vi "scope_viewer.vi"() -> ()   [LabVIEW 2019]
uses:
  <instrlib>/niScope/Controls/niScope trigger source.ctl
  <instrlib>/niScope/Controls/niScope trigger coupling.ctl
  <instrlib>/niScope/Controls/niScope trigger slope.ctl
  <instrlib>/niScope/Controls/niScope vertical coupling.ctl
  <vilib>/Waveform/WDTOps.llb/WDT Align Waveform Timestamps DBL.vi
  <vilib>/Waveform/WDTFileIO.llb/Export Waveform To Spreadsheet File.vi
  <instrlib>/niScope/Acquire/Fetch/niScope Fetch WDT.vi
  <instrlib>/niScope/Configure/Trigger/niScope Configure Trigger Edge.vi
  <vilib>/regexp/Match Regular Expression.xnode
panel:
  in  "Tab Control":T1(tab)
  in  "C1 vertical coupling":T2=1 caption="vertical coupling" items=["AC", "DC", "Ground"]
  in  "C1 probe attenuation":dbl=1.0 caption="probe attenuation" format="%.1f"
  in  "C1 vertical range":dbl=5.0 caption="vertical range" min=0.1 max=5.0 step=0.1 format="%.2f"
  in  "C1 vertical offset":dbl caption="vertical offset" format="%.4f"
  in  "C1 enabled":bool=TRUE caption="Enabled?"
  in  "C1 maximum input frequency":dbl caption="max input frequency" format="%.2f"
  in  "C1 input impedance":u32(ring) caption="input impedance" items=["1 mega ohm"=0, "50 ohms"=2]
  in  "C2 enabled":bool=TRUE caption="Enabled?"
  in  "C2 input impedance":u32(ring) caption="input impedance" items=["1 mega ohm"=0, "50 ohms"=2]
  in  "C2 maximum input frequency":dbl caption="max input frequency" format="%.2f"
  in  "C2 vertical coupling":T2=1 caption="vertical coupling" items=["AC", "DC", "Ground"]
  in  "C2 probe attenuation":dbl=1.0 caption="probe attenuation" format="%.1f"
  in  "C2 vertical range":dbl=5.0 caption="vertical range" min=0.1 max=5.0 step=0.1 format="%.2f"
  in  "C2 vertical offset":dbl caption="vertical offset" format="%.4f"
  in  "Num Trace":dbl=1.0 min=1.0 step=1.0
  in  "Summed/Average":u16(ring) items=["Average", "Summed"]
  in  "Trigger delay":dbl caption="trigger delay" format="%.4f"
  in  "Trigger slope":T3 items=["Positive", "Negative"]
  in  "Trigger level":dbl=0.5
  in  "Trigger coupling":T4=1 caption="C1 trigger coupling" items=["AC"=0, "DC"=1, "HF Reject"=3, "LF Reject"=4, "AC Plus HF Reject"=1001]
  in  "Trigger source":T5="0" caption="Source"
  out "Aqusition Time / ms":u32
  out "Aquisition Frequency / Hz":dbl
  in  "tmax (\\mu s)":dbl
  in  "Samples":i64(ring) items=["500 S"=500, "1 kS"=1000, "5 kS"=5000, "10 kS"=10000, "100 kS"=100000, "500 kS"=500000, "1 MS"=1000000, "2.5 MS"=2500000, "5MS"=5000000, "10 MS"=10000000, "20 MS"=20000000]
  in  "Scope Channel":refnum<k15> caption="resource name"
  in  "stop":bool
  in  "Enforce realtime":bool=TRUE caption="enforce realtime"
  in  "Save Scope Conditions":bool
  in  "Load Scope Conditions":bool
  in  "waveforms out 2":waveform(dbl)[](array[waveform])
  in  "Tab Control 2":T6(tab)
  in  "Tab Control 3":enum32{"Channel 1", "Channel 2"}(tab)
  out "Channel 1 Raw":waveform(dbl)(graph)
  out "Channel 2 Raw":waveform(dbl)(graph)
  in  "Tab Control 4":enum32{"Channel 1", "Channel 2"}(tab)
  out "Channel 1 RT avg":waveform(dbl)(graph)
  out "Channel 2 RT avg":waveform(dbl)(graph)
  in  "Tab Control 5":enum32{"Channel 1", "Channel 2"}(tab)
  out "Channel 1 summed":waveform(dbl)(graph)
  out "Channel 2 summed":waveform(dbl)(graph)
  # "Scope Controls"
  # "Channel Enabled?"
  # "Channel Enabled?"
  # "Scope Conditions:"
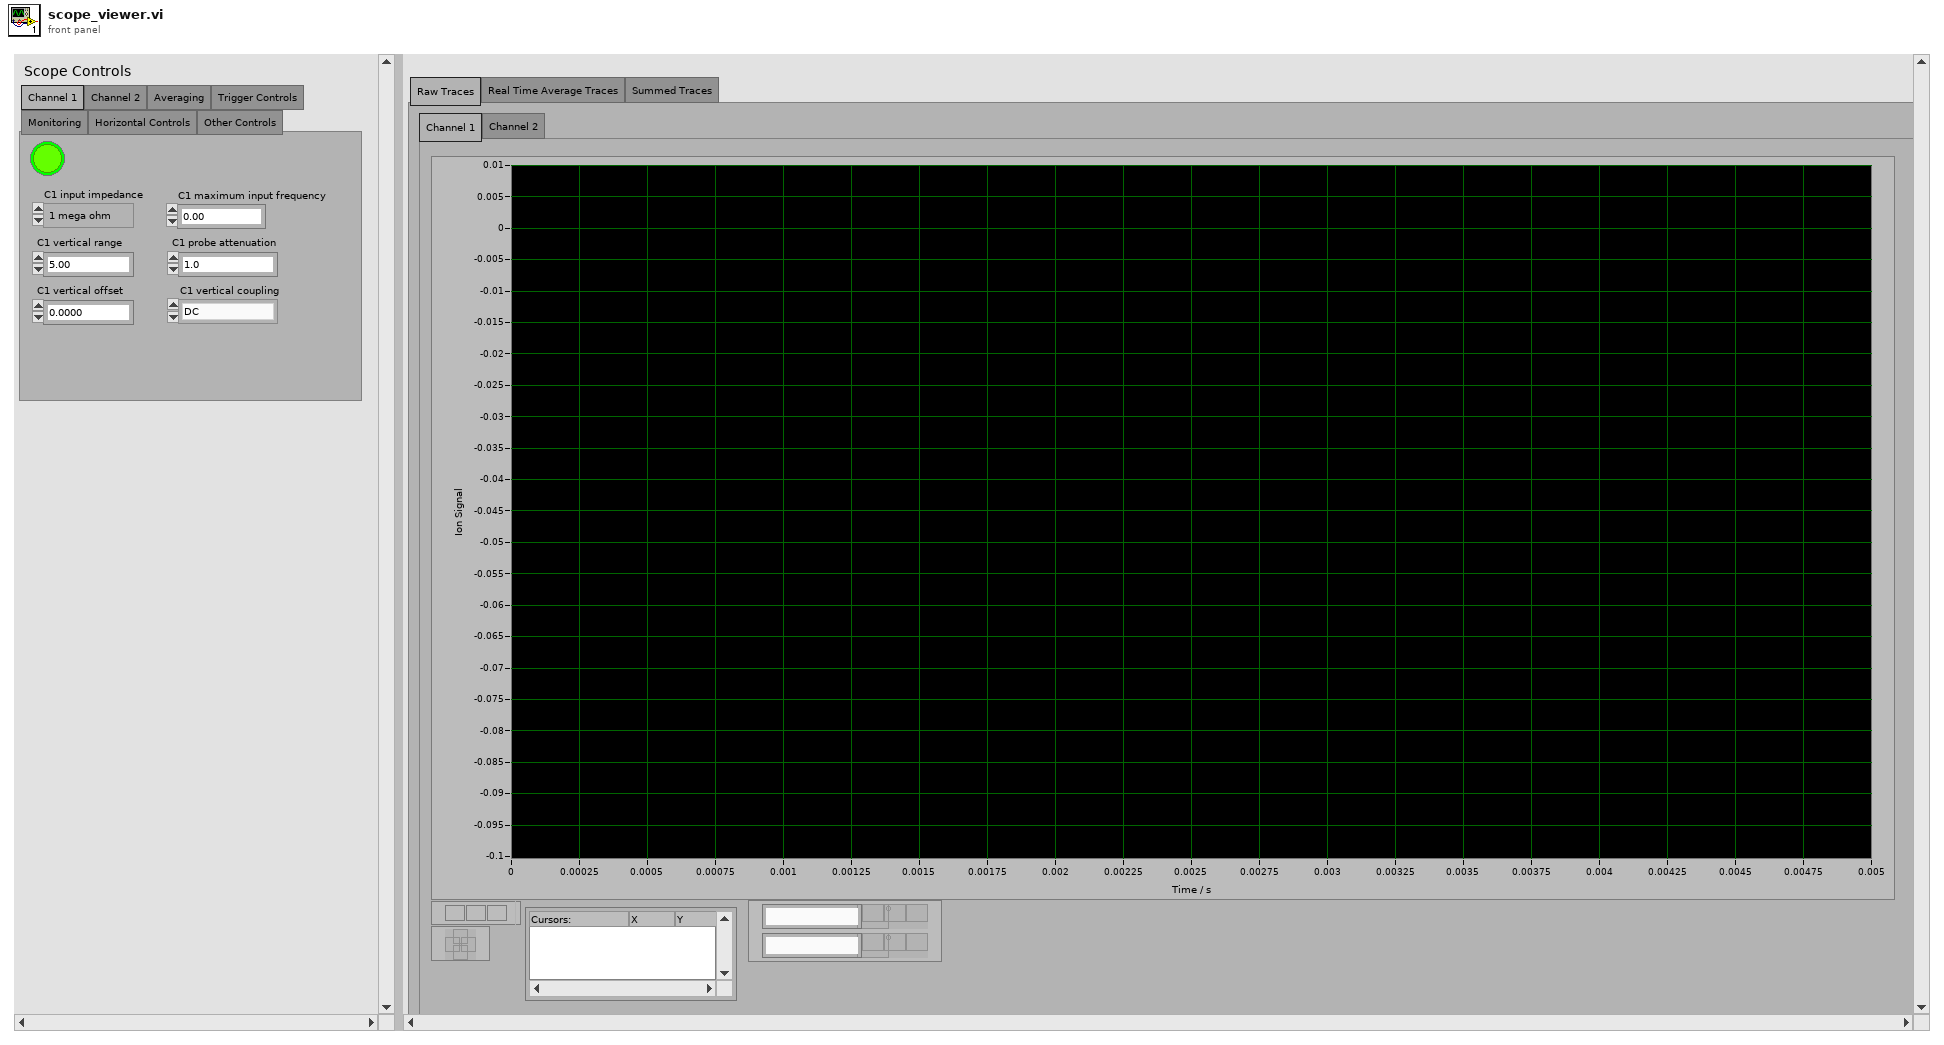
[diagram p1: front panel]
types:
  T1 = enum32{"Channel 1", "Channel 2", "Averaging", "Trigger Controls", "Monitoring", "Horizontal Controls", "Other Controls"}
  T2 = typedef "niScope vertical coupling.ctl" = i32
  T3 = typedef "niScope trigger slope.ctl" = i32
  T4 = typedef "niScope trigger coupling.ctl" = u16
  T5 = typedef "niScope trigger source.ctl" = string
  T6 = enum32{"Raw Traces", "Real Time Average Traces", "Summed Traces"}
  T7 = cluster{"C2 vertical offset":dbl, "C2 vertical range":dbl, "C2 probe attenuation":dbl, "C2 vertical coupling":T2, "C2 maximum input frequency":dbl, "C2 input impedance":u32, "C2 enabled":bool, "C1 input impedance":u32, "C1 maximum input frequency":dbl, "C1 enabled":bool, "C1 vertical offset":dbl, "C1 vertical range":dbl, "C1 probe attenuation":dbl, "C1 vertical coupling":T2, "Samples":i64, "tmax (\\mu s) ":dbl, "Trigger source":T5, "Trigger coupling":T4, "Trigger level":dbl, "Trigger slope":T3, "Trigger delay":dbl, "Enforce realtime":bool, "Aquisition Frequency / Hz":dbl, "Aqusition Time / ms":u32, "Scope Channel":refnum<k15>}
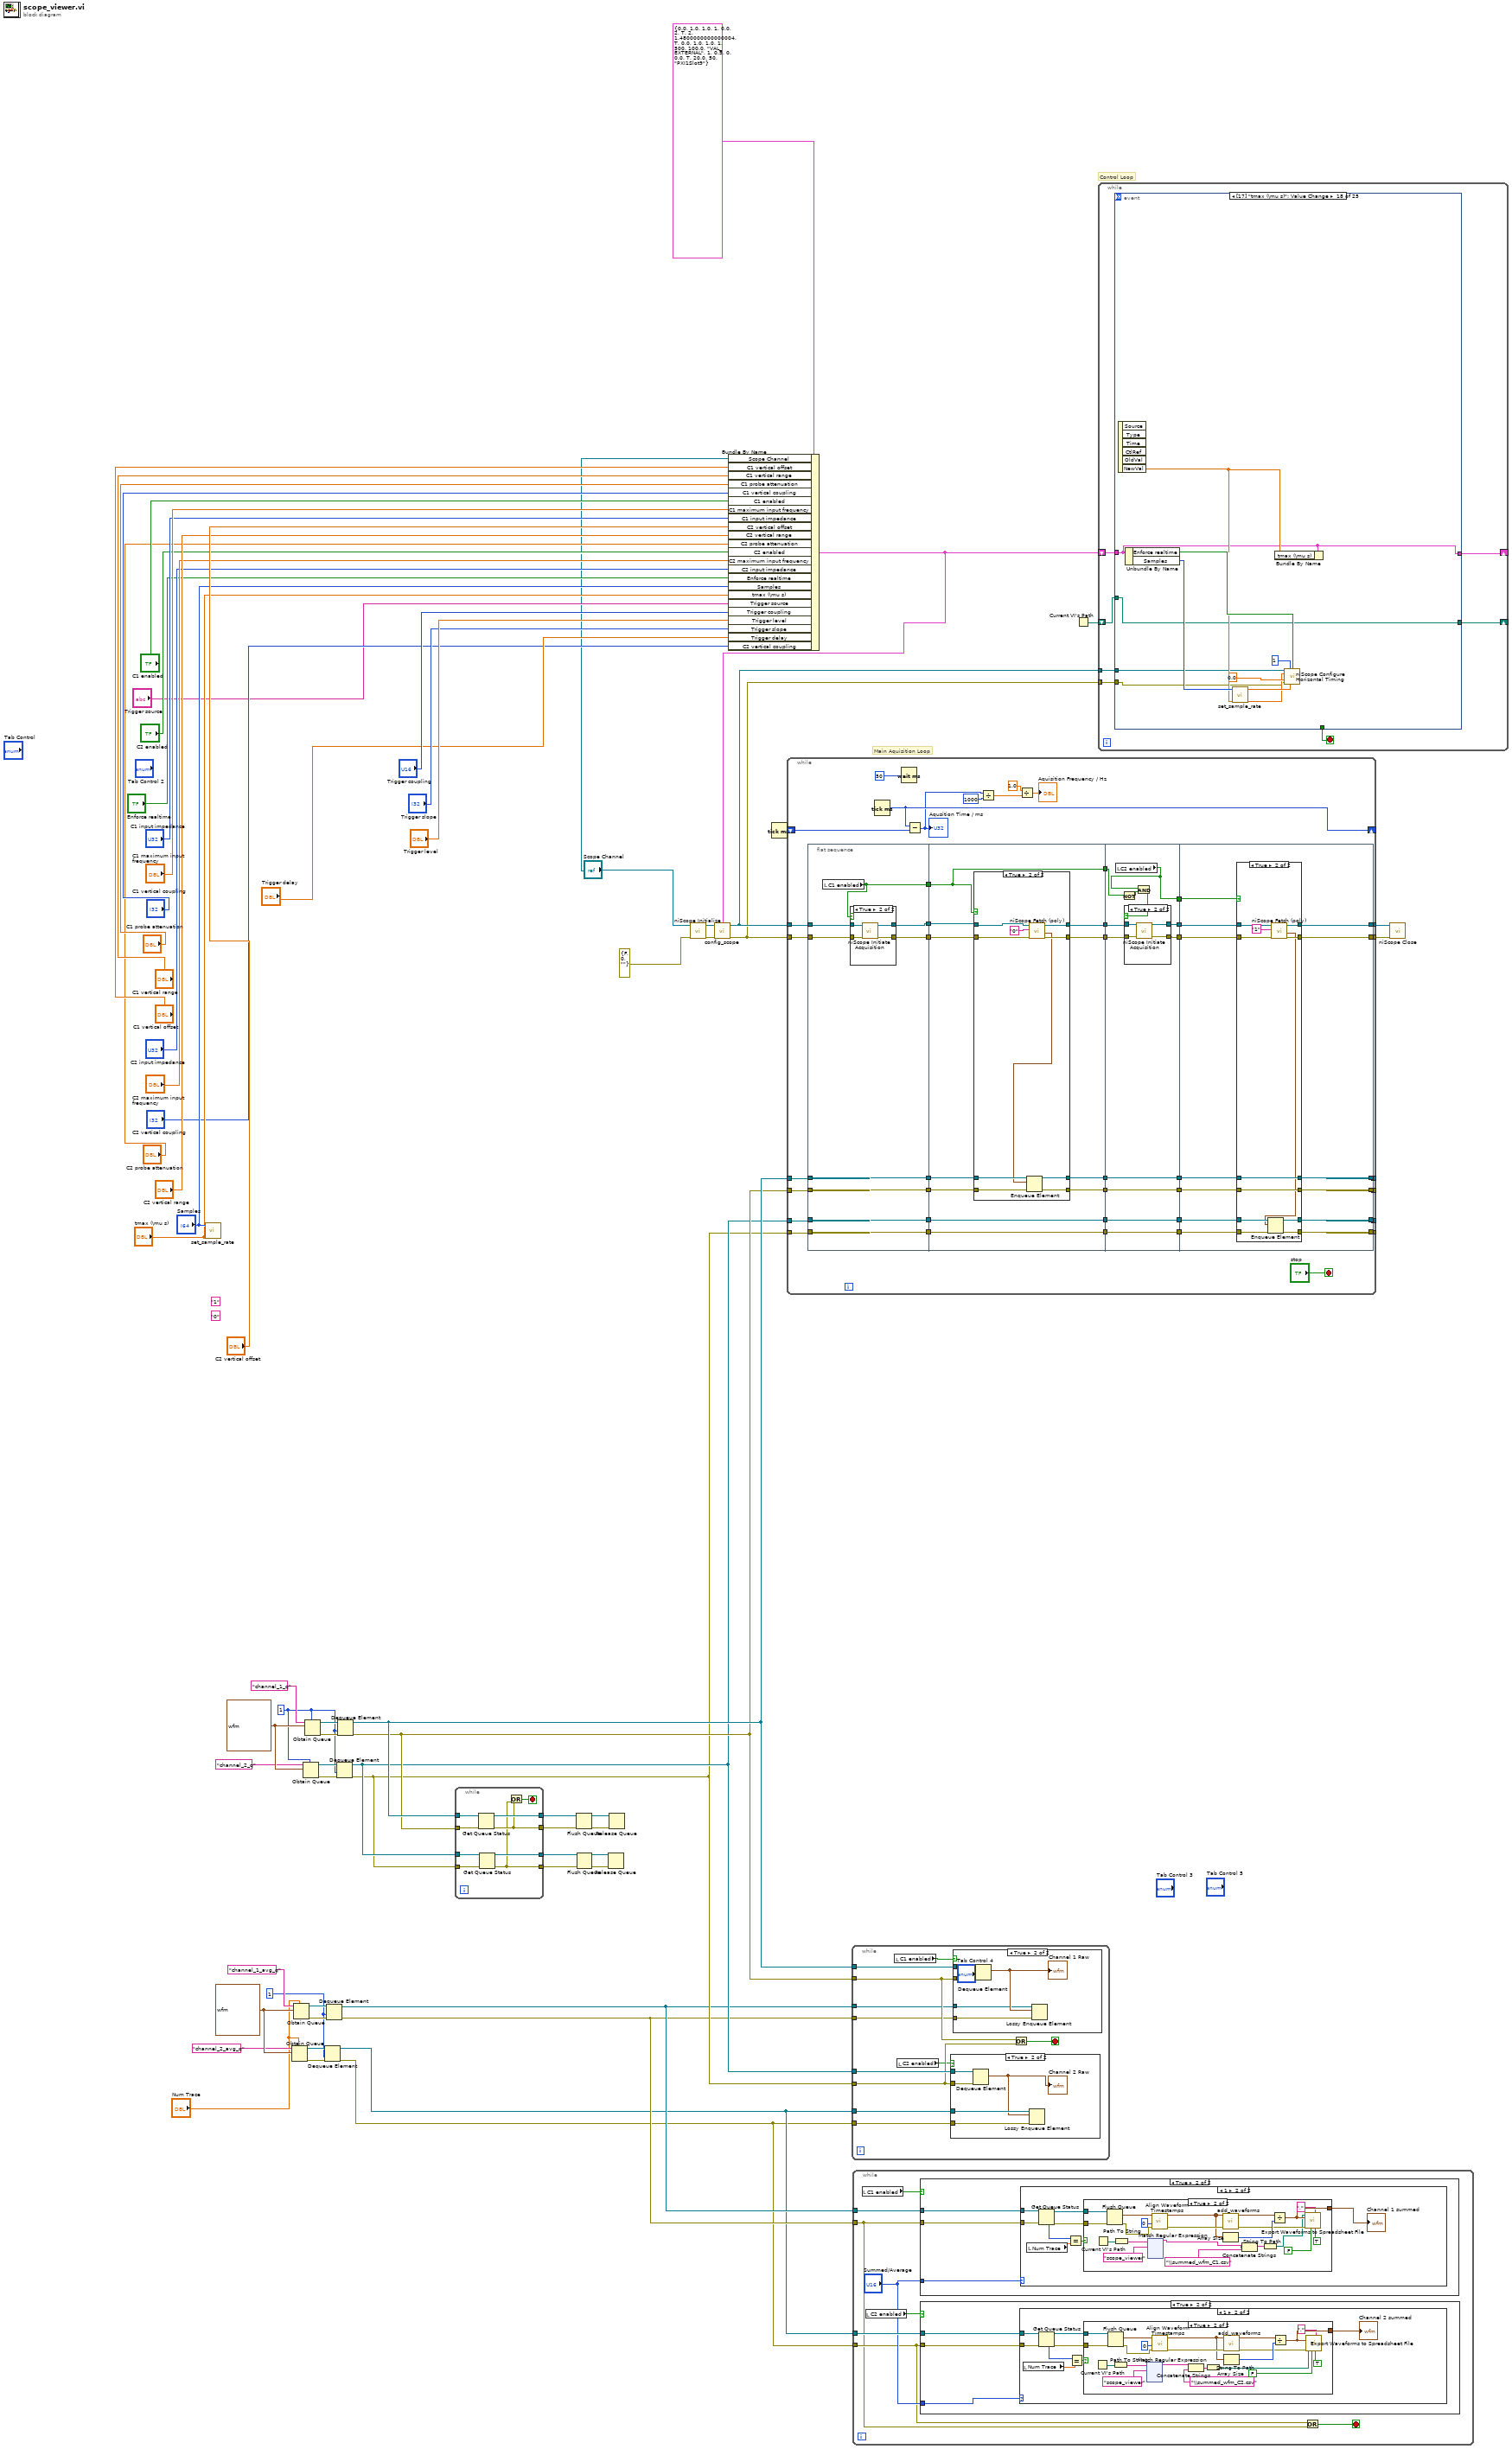
[diagram p0: block diagram]
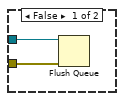
[diagram p2: hidden frame]
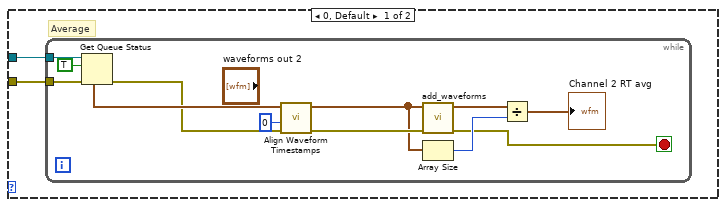
[diagram p3: hidden frame]
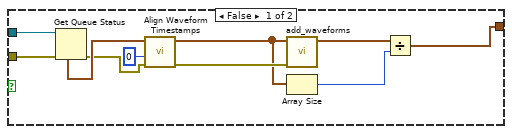
[diagram p4: hidden frame]
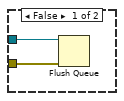
[diagram p5: hidden frame]
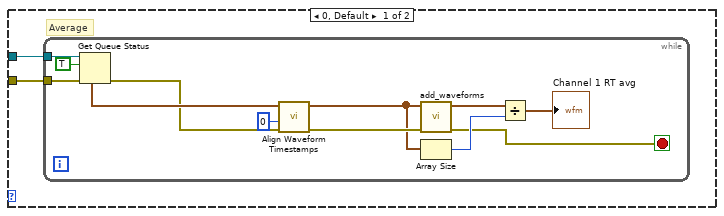
[diagram p6: hidden frame]
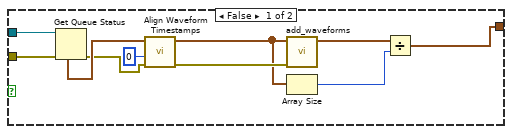
[diagram p7: hidden frame]
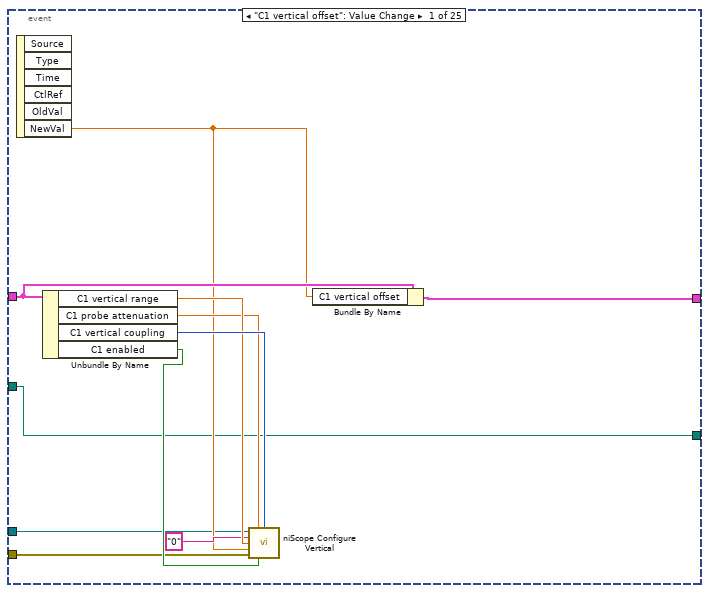
[diagram p8: hidden frame]
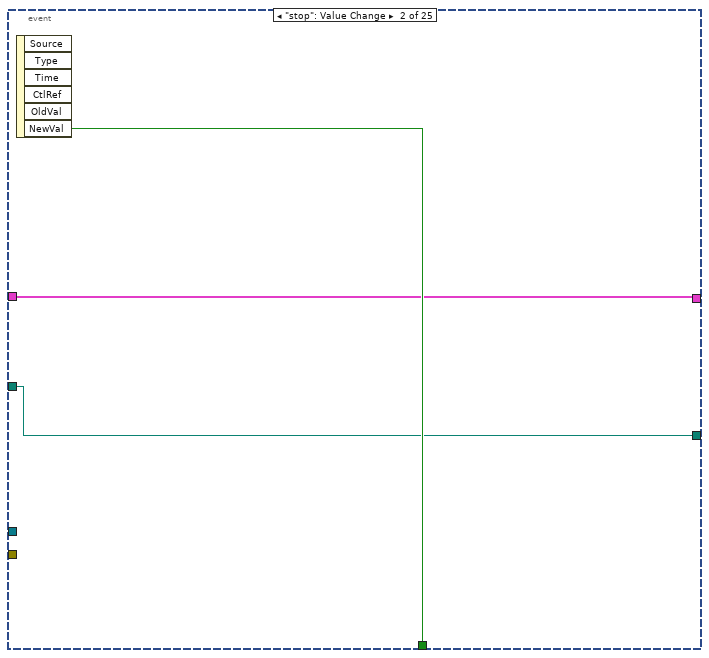
[diagram p9: hidden frame]
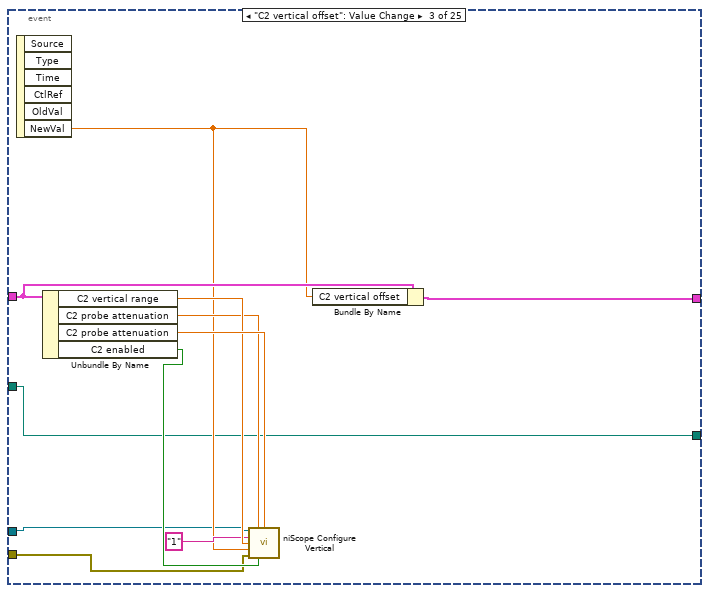
[diagram p10: hidden frame]
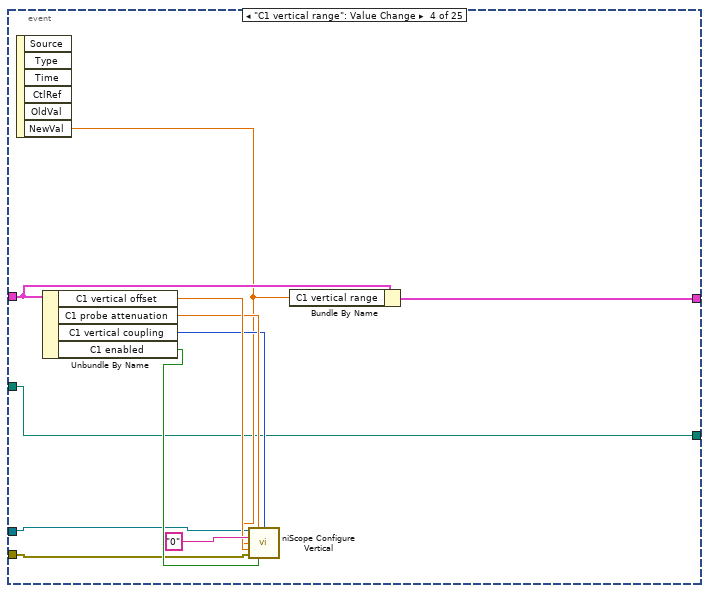
[diagram p11: hidden frame]
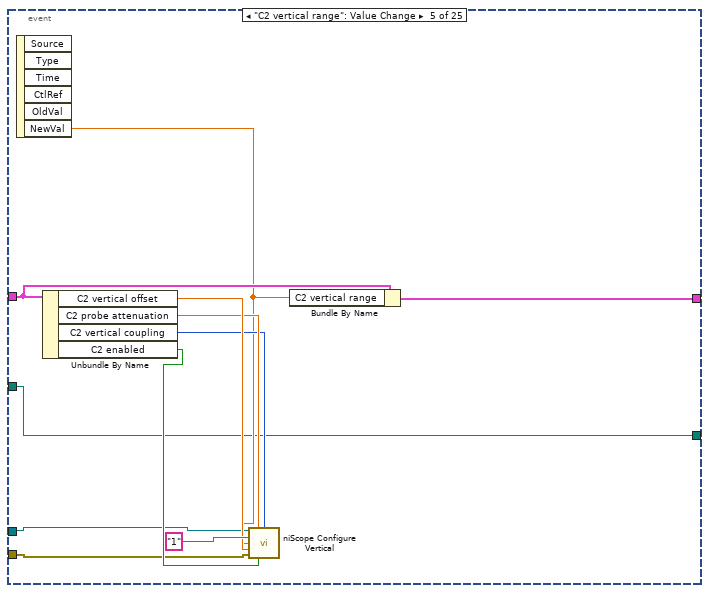
[diagram p12: hidden frame]
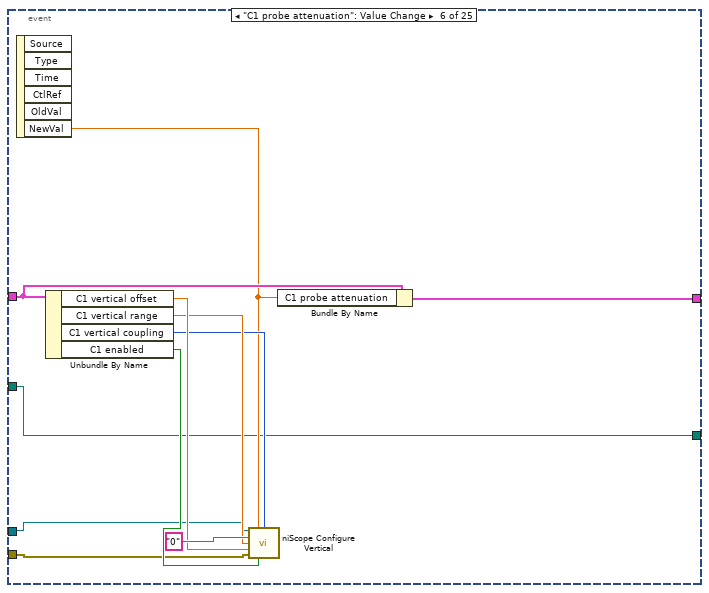
[diagram p13: hidden frame]
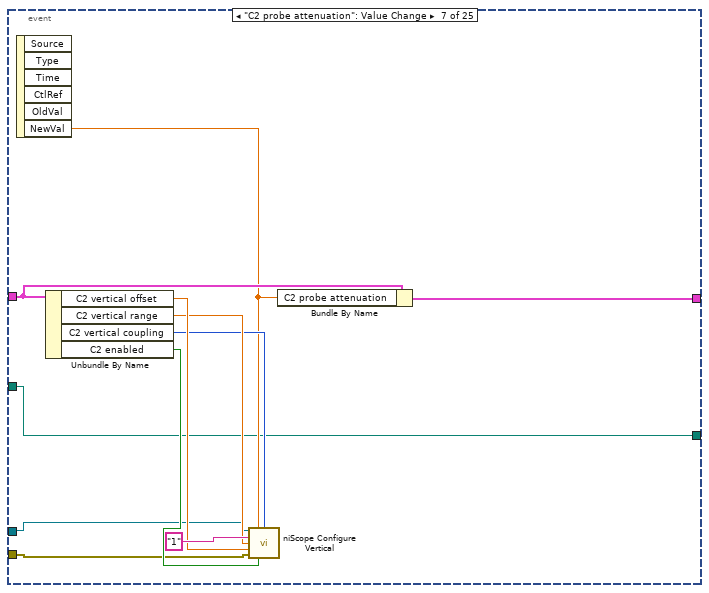
[diagram p14: hidden frame]
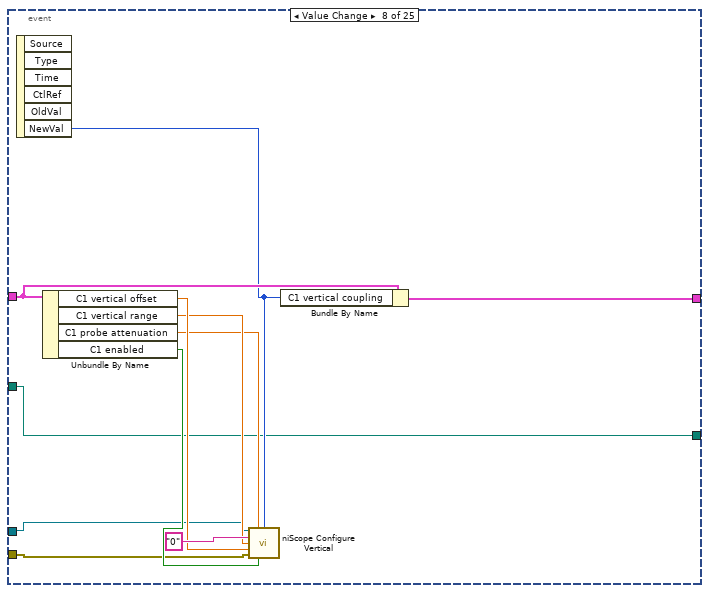
[diagram p15: hidden frame]
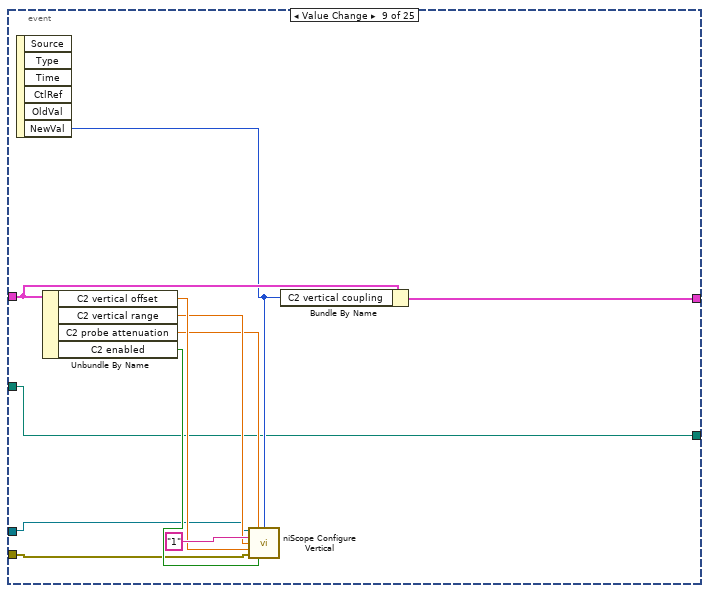
[diagram p16: hidden frame]
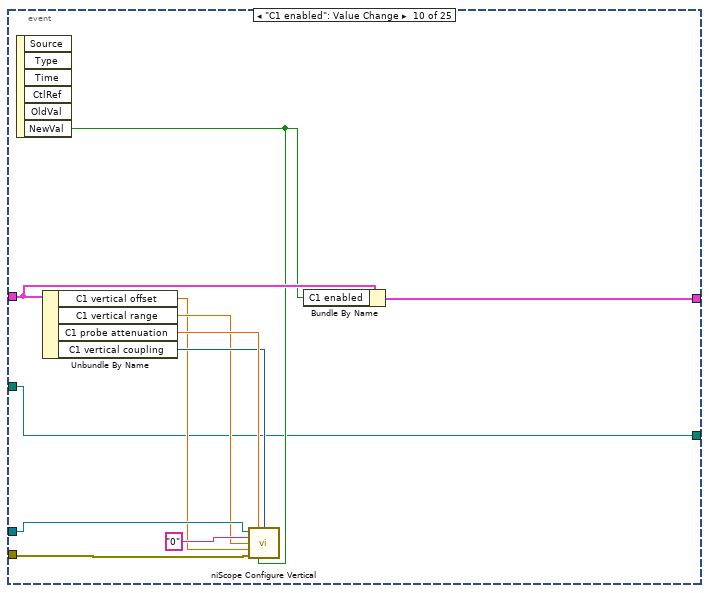
[diagram p17: hidden frame]
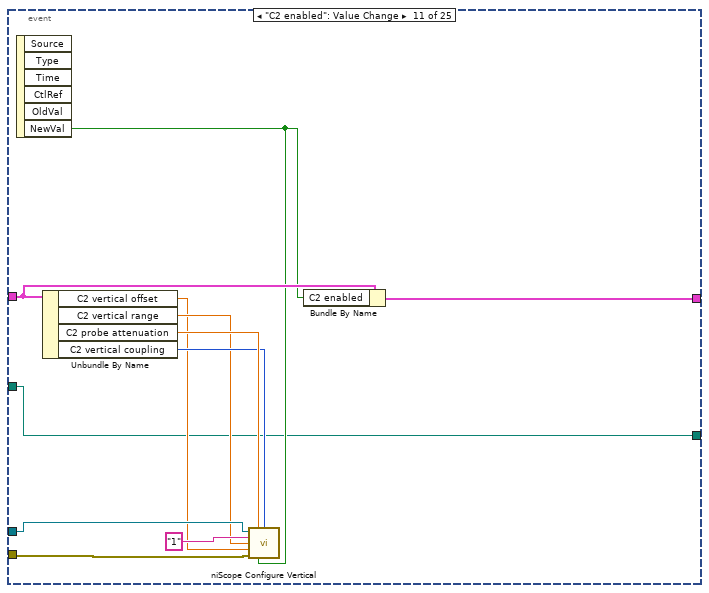
[diagram p18: hidden frame]
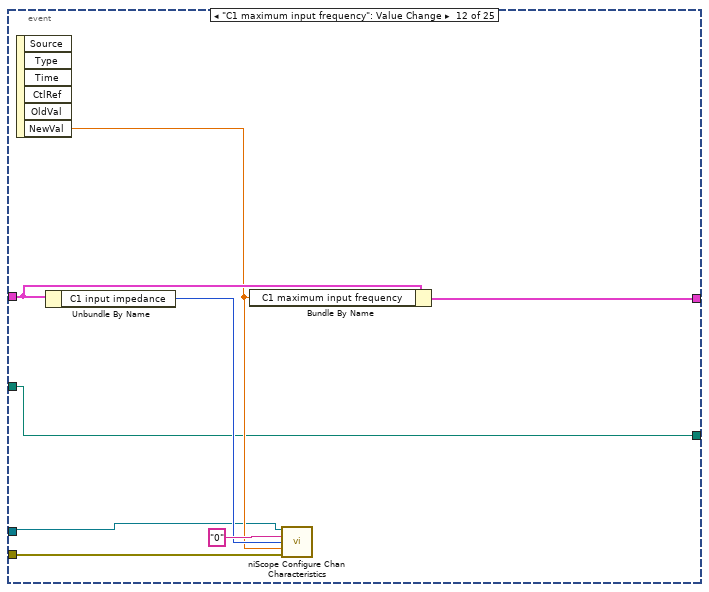
[diagram p19: hidden frame]
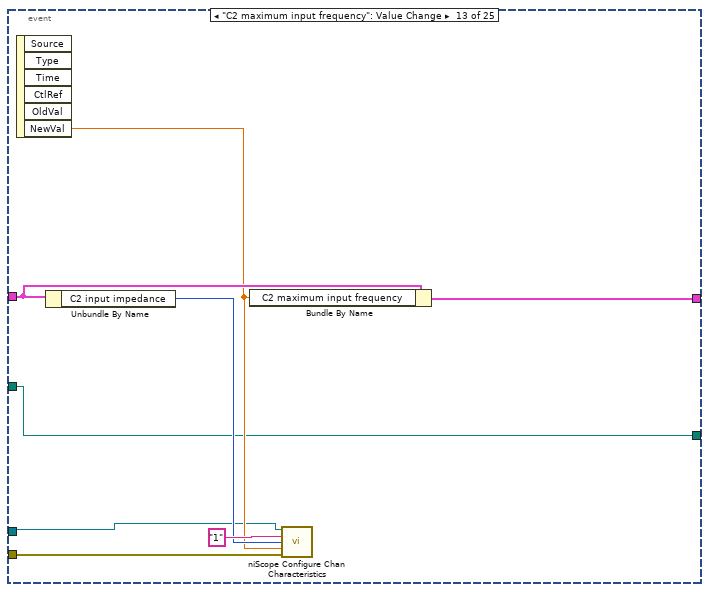
[diagram p20: hidden frame]
diagram:
  w6 = 1 ("max queue size (-1, unlimited)")
  w9 = waveform(dbl) {"t0"=timestamp(0 s since 1904-01-01), "dt"=1.0, "Y"=[]} ("wfm")
  w55 = 1 ("max queue size (-1, unlimited)")
  w58 = waveform(dbl) {"t0"=timestamp(0 s since 1904-01-01), "dt"=1.0, "Y"=[]} ("wfm")
  (unwired) "1" ("channels")
  (unwired) "0" ("index")
  # "Control Loop"
  # "Main Aquisition Loop"
  n1 = call "set_sample_rate.vi"("t max / us"="tmax (\\mu s)", "Samples"="Samples") -> ()  [unwired: 8 in, 2 out]
  n2 = Obtain Queue(max queue size (-1, unlimited)="Num Trace", name (unnamed)="channel_2_avg_q", element data type=w9) -> (queue out=w11:refnum<queue>, error out=w10:errorcluster)  [unwired: 2 in, 1 out]
  n3 = Obtain Queue(max queue size (-1, unlimited)="Num Trace", name (unnamed)="channel_1_avg_q", element data type=w9) -> (queue out=w13:refnum<queue>, error out=w12:errorcluster)  [unwired: 2 in, 1 out]
  n4 = Obtain Queue(max queue size (-1, unlimited)=w55, name (unnamed)="channel_2_q", element data type=w58) -> (queue out=w60:refnum<queue>, error out=w59:errorcluster)  [unwired: 2 in, 1 out]
  n5 = Obtain Queue(max queue size (-1, unlimited)=w55, name (unnamed)="channel_1_q", element data type=w58) -> (queue out=w62:refnum<queue>, error out=w61:errorcluster)  [unwired: 2 in, 1 out]
  n6 = Dequeue Element(queue=w11, timeout in ms (-1)=w6, error in (no error)=w10) -> (queue out=w3:refnum<queue>, error out=w2:errorcluster)  [unwired: 2 out]
  n7 = Dequeue Element(queue=w13, timeout in ms (-1)=w6, error in (no error)=w12) -> (queue out=w5:refnum<queue>, error out=w4:errorcluster)  [unwired: 2 out]
  n8 = Dequeue Element(queue=w60, timeout in ms (-1)=w55, error in (no error)=w59) -> (queue out=w48:refnum<queue>, error out=w47:errorcluster)  [unwired: 2 out]
  n9 = Dequeue Element(queue=w62, timeout in ms (-1)=w55, error in (no error)=w61) -> (queue out=w50:refnum<queue>, error out=w49:errorcluster)  [unwired: 2 out]
  n10 = while {
    tunnel: w50 -> [w76]
    tunnel: w49 -> [w75]
    tunnel: w48 -> [w74]
    tunnel: w47 -> [w73]
    tunnel: [w72] -> w54
    tunnel: [w70] -> w53
    tunnel: [w71] -> w52
    tunnel: [w69] -> w51
    stop <- w68 stop-if-true
    n11 = Get Queue Status(queue=w76, error in (no error)=w75) -> (queue out=w72:refnum<queue>, error out=w70:errorcluster)  [unwired: 1 in, 6 out]
    n12 = Get Queue Status(queue=w74, error in (no error)=w73) -> (queue out=w71:refnum<queue>, error out=w69:errorcluster)  [unwired: 1 in, 6 out]
    n13 = Or(x=w70, y=w69) -> (x .or. y?=w68:bool)
  }
  n14 = Flush Queue(queue=w54, error in (no error)=w53) -> (queue out=w17:refnum<queue>, error out=w16:errorcluster)  [unwired: 1 out]
  n15 = Flush Queue(queue=w52, error in (no error)=w51) -> (queue out=w15:refnum<queue>, error out=w14:errorcluster)  [unwired: 1 out]
  n16 = Release Queue(queue=w15, error in (no error)=w14) -> ()  [unwired: 1 in, 3 out]
  n17 = Release Queue(queue=w17, error in (no error)=w16) -> ()  [unwired: 1 in, 3 out]
  n18 = call <instrlib>:"niScope Initialize.vi"("resource name"="Scope Channel", "error in"=errorcluster {"status"=FALSE, "code"=0, "source"=""}) -> ("instrument handle"=w22:refnum<k15>, "error out"=w21:errorcluster)  [unwired: 12 in]
  n19 = Bundle By Name(cluster=T7 {"C2 vertical offset"=0.0, "C2 vertical range"=1.0, "C2 probe attenuation"=1.0, "C2 vertical coupling"=1, "C2 maximum input frequency"=0.0, "C2 input impedance"=2, "C2 enabled"=TRUE, "C1 input impedance"=2, "C1 maximum input frequency"=1.4800000000000004, "C1 enabled"=TRUE, "C1 vertical offset"=0.0, "C1 vertical range"=1.0, "C1 probe attenuation"=1.0, "C1 vertical coupling"=1, "Samples"=500, "tmax (\\mu s) "=100.0, "Trigger source"="VAL_EXTERNAL", "Trigger coupling"=1, "Trigger level"=0.5, "Trigger slope"=0, "Trigger delay"=0.0, "Enforce realtime"=TRUE, "Aquisition Frequency / Hz"=20.0, "Aqusition Time / ms"=50, "Scope Channel"="PXI1Slot9"} ("Cluster"), "Scope Channel"=w22, "C1 vertical offset"="C1 vertical offset", "C1 vertical range"="C1 vertical range", "C1 probe attenuation"="C1 probe attenuation", "C1 vertical coupling"="C1 vertical coupling", "C1 enabled"="C1 enabled", "C1 maximum input frequency"="C1 maximum input frequency", "C1 input impedance"="C1 input impedance", "C2 vertical offset"="C2 vertical offset", "C2 vertical range"="C2 vertical range", "C2 probe attenuation"="C2 probe attenuation", "C2 enabled"="C2 enabled", "C2 maximum input frequency"="C2 maximum input frequency", "C2 input impedance"="C2 input impedance", "Enforce realtime"="Enforce realtime", "Samples"="Samples", "tmax (\\mu s)"="tmax (\\mu s)", "Trigger source"="Trigger source", "Trigger coupling"="Trigger coupling", "Trigger level"="Trigger level", "Trigger slope"="Trigger slope", "Trigger delay"="Trigger delay", "C2 vertical coupling"="C2 vertical coupling") -> (w20:T7)
  n20 = call "config_scope.vi"("instrument handle"=w22, "Scope Config Data"=w20, "error in"=w21) -> ("instrument handle out"=w19:refnum<k15>, "error out"=w18:errorcluster)  [unwired: 11 in]
  n21 = Tick Count (ms)() -> (millisecond timer value=w66:u32)
  n22 = while {
    shift-right: [w114] -> _
    shift-left: w66 -> [w117]
    tunnel: [w110] -> w64
    tunnel: [w109] -> w63
    tunnel: w50 -> [w107]
    tunnel: w49 -> [w106]
    tunnel: [w105] -> _
    tunnel: [w104] -> _
    tunnel: w48 -> [w103]
    tunnel: w47 -> [w102]
    tunnel: [w101] -> _
    tunnel: [w100] -> _
    tunnel: w19 -> [w93]
    tunnel: w18 -> [w92]
    stop <- "stop" stop-if-true
    n23 = flat-sequence {
      tunnel: w102 -> [w124]
      tunnel: w103 -> [w125]
      tunnel: w106 -> [w126]
      tunnel: w107 -> [w127]
      tunnel: [w127] -> w99
      tunnel: [w126] -> w98
      tunnel: [w125] -> w97
      tunnel: [w124] -> w96
      tunnel: [w121] -> w95
      tunnel: [w120] -> w94
      tunnel: w93 -> [w123]
      tunnel: w92 -> [w122]
      tunnel: [w119] -> w91
      tunnel: [w144] -> w90
      tunnel: [w143] -> w88
      tunnel: [w140] -> w87
      tunnel: [w139] -> w85
      tunnel: [w138] -> w83
      tunnel: [w137] -> w81
      tunnel: w99 -> [w142]
      tunnel: w98 -> [w141]
      tunnel: w97 -> [w138]
      tunnel: w96 -> [w137]
      tunnel: w95 -> [w136]
      tunnel: w94 -> [w135]
      tunnel: w91 -> [w134]
      tunnel: [w134] -> w77
      tunnel: w90 -> [w167]
      tunnel: [w169] -> w89
      tunnel: w88 -> [w166]
      tunnel: w87 -> [w173]
      tunnel: [w173] -> w86
      tunnel: w85 -> [w172]
      tunnel: [w172] -> w84
      tunnel: w83 -> [w171]
      tunnel: [w171] -> w82
      tunnel: w81 -> [w170]
      tunnel: [w170] -> w80
      tunnel: [w168] -> w79
      tunnel: [w164] -> w78
      tunnel: w77 -> [w162]
      tunnel: w89 -> [w192]
      tunnel: [w190] -> w110
      tunnel: [w189] -> w109
      tunnel: w86 -> [w188]
      tunnel: w84 -> [w187]
      tunnel: [w186] -> w105
      tunnel: [w185] -> w104
      tunnel: w82 -> [w184]
      tunnel: w80 -> [w183]
      tunnel: [w182] -> w101
      tunnel: [w181] -> w100
      tunnel: w79 -> [w191]
      tunnel: w78 -> [w180]
      frame #0 {
        n24 = local read "C1 enabled"() -> (w119:bool)
        n25 = case shown="True" w119 {
          tunnel: w123 -> [w129 w133]
          tunnel: w122 -> [w128 w132]
          tunnel: [w129 w131] -> w121
          tunnel: [w128 w130] -> w120
          frame False {
          }
          frame True {
            n26 = call <instrlib>:"niScope Initiate Acquisition.vi"("instrument handle"=w133, "error in"=w132) -> ("instrument handle out"=w131:refnum<k15>, "error out"=w130:errorcluster)  [unwired: 12 in]
          }
        }
      }
      frame #1 {
        n27 = case shown="True" w134 {
          tunnel: w136 -> [w146 w161]
          tunnel: w135 -> [w145 w160]
          tunnel: [w146 w159] -> w144
          tunnel: [w145 w158] -> w143
          tunnel: w142 -> [w151 w156]
          tunnel: w141 -> [w148 w155]
          tunnel: [w150 w153] -> w140
          tunnel: [w149 w152] -> w139
          frame False {
            n28 = Enqueue Element(queue=w151, element=waveform(dbl) {"t0"=timestamp(0 s since 1904-01-01), "dt"=1.0, "Y"=[]}, error in (no error)=w148) -> (queue out=w150:refnum<queue>, error out=w149:errorcluster)  [unwired: 1 in, 1 out]
          }
          frame True {
            n29 = call-poly <instrlib>:"niScope Fetch (poly).vi"("error in"=w160, "channels"="0", "instrument handle"=w161) -> ("error out"=w158:errorcluster, "wfm"=w154:waveform(dbl), "instrument handle out"=w159:refnum<k15>)  [unwired: 5 in, 1 out]
            n30 = Enqueue Element(queue=w156, element=w154, error in (no error)=w155) -> (queue out=w153:refnum<queue>, error out=w152:errorcluster)  [unwired: 1 in, 1 out]
          }
        }
      }
      frame #2 {
        n31 = local read "C2 enabled"() -> (w164:bool)
        n32 = Not(x=w162) -> (.not. x?=w163:bool)
        n33 = And(x=w164, y=w163) -> (x .and. y?=w165:bool)
        n34 = case shown="True" w165 {
          tunnel: w167 -> [w175 w179]
          tunnel: w166 -> [w174 w178]
          tunnel: [w175 w177] -> w169
          tunnel: [w174 w176] -> w168
          frame False {
          }
          frame True {
            n35 = call <instrlib>:"niScope Initiate Acquisition.vi"("instrument handle"=w179, "error in"=w178) -> ("instrument handle out"=w177:refnum<k15>, "error out"=w176:errorcluster)  [unwired: 12 in]
          }
        }
      }
      frame #3 {
        n36 = case shown="True" w180 {
          tunnel: w192 -> [w194 w213]
          tunnel: w191 -> [w193 w212]
          tunnel: [w194 w211] -> w190
          tunnel: [w193 w210] -> w189
          tunnel: w188 -> [w201 w208]
          tunnel: w187 -> [w200 w207]
          tunnel: [w201 w208] -> w186
          tunnel: [w200 w207] -> w185
          tunnel: w184 -> [w199 w206]
          tunnel: w183 -> [w197 w205]
          tunnel: [w198 w203] -> w182
          tunnel: [w196 w202] -> w181
          frame False {
            n37 = Enqueue Element(queue=w199, element=waveform(dbl) {"t0"=timestamp(0 s since 1904-01-01), "dt"=1.0, "Y"=[]}, error in (no error)=w197) -> (queue out=w198:refnum<queue>, error out=w196:errorcluster)  [unwired: 1 in, 1 out]
          }
          frame True {
            n38 = call-poly <instrlib>:"niScope Fetch (poly).vi"("error in"=w212, "channels"="1", "instrument handle"=w213) -> ("error out"=w210:errorcluster, "wfm"=w204:waveform(dbl), "instrument handle out"=w211:refnum<k15>)  [unwired: 5 in, 1 out]
            n39 = Enqueue Element(queue=w206, element=w204, error in (no error)=w205) -> (queue out=w203:refnum<queue>, error out=w202:errorcluster)  [unwired: 1 in, 1 out]
          }
        }
      }
    }
    n40 = Tick Count (ms)() -> (millisecond timer value=w114:u32)
    n41 = Wait (ms)(milliseconds to wait=u32 50) -> ()  [unwired: 1 out]
    n42 = Subtract(x=w114, y=w117) -> (x-y=w108:u32)
    "Aqusition Time / ms" <- w108
    n43 = Divide(x=w108, y=u32 1000) -> (x/y=w115:dbl)
    n44 = Divide(x=1.0, y=w115) -> (x/y=→"Aquisition Frequency / Hz":dbl)
  }
  n45 = while {
    tunnel: w50 -> [w224]
    tunnel: w49 -> [w221]
    tunnel: w48 -> [w218]
    tunnel: w47 -> [w217]
    tunnel: w5 -> [w220]
    tunnel: w4 -> [w219]
    tunnel: w3 -> [w215]
    tunnel: w2 -> [w214]
    stop <- w222 stop-if-true
    n46 = local read "C1 enabled"() -> (w223:bool)
    n47 = local read "C2 enabled"() -> (w216:bool)
    n48 = case shown="True" w216 {
      tunnel: w218 -> [w226 w231]
      tunnel: w217 -> [w225 w230]
      tunnel: w215 -> [_ w229]
      tunnel: w214 -> [_ w228]
      frame False {
        n49 = Flush Queue(queue=w226, error in (no error)=w225) -> ()  [unwired: 3 out]
      }
      frame True {
        n50 = Dequeue Element(queue=w231, error in (no error)=w230) -> (element=w227:waveform(dbl))  [unwired: 1 in, 3 out]
        "Channel 2 Raw" <- w227
        n51 = Lossy Enqueue Element(queue=w229, element=w227, error in (no error)=w228) -> ()  [unwired: 4 out]
      }
    }
    n52 = case shown="True" w223 {
      tunnel: w224 -> [w233 w238]
      tunnel: w221 -> [w232 w237]
      tunnel: w220 -> [_ w235]
      tunnel: w219 -> [_ w234]
      frame False {
        n53 = Flush Queue(queue=w233, error in (no error)=w232) -> ()  [unwired: 3 out]
      }
      frame True {
        n54 = Dequeue Element(queue=w238, error in (no error)=w237) -> (element=w236:waveform(dbl))  [unwired: 1 in, 3 out]
        "Channel 1 Raw" <- w236
        n55 = Lossy Enqueue Element(queue=w235, element=w236, error in (no error)=w234) -> ()  [unwired: 4 out]
      }
    }
    n56 = Or(x=w221, y=w217) -> (x .or. y?=w222:bool)
  }
  n57 = while {
    tunnel: w5 -> [w245]
    tunnel: w4 -> [w239]
    tunnel: w3 -> [w244]
    tunnel: w2 -> [w240]
    stop <- w241 stop-if-true
    n58 = local read "C1 enabled"() -> (w246:bool)
    n59 = local read "C2 enabled"() -> (w242:bool)
    n60 = case shown="True" w246 {
      tunnel: w245 -> [w420 w422]
      tunnel: w239 -> [w419 w421]
      tunnel: "Summed/Average" -> [_ w423]
      frame False {
        n61 = Flush Queue(queue=w420, error in (no error)=w419) -> ()  [unwired: 3 out]
      }
      frame True {
        n62 = case shown="1" w423 {
          tunnel: w422 -> [w425 w444]
          tunnel: w421 -> [w424 w445]
          frame 0, Default {
            # "Average"
            n63 = while {
              tunnel: w425 -> [w437]
              tunnel: w424 -> [w436]
              stop <- w428 stop-if-true
              n64 = Get Queue Status(queue=w437, return elements? (F)=TRUE, error in (no error)=w436) -> (error out=w434:errorcluster, elements=w435:waveform(dbl)[])  [unwired: 6 out]
              n65 = call-poly <vilib>:"Align Waveform Timestamps.vi"("error in (no error)"=w434, "index"=0, "waveforms in"=w435) -> ("error out"=w433:errorcluster, "waveforms out"=w430:waveform(dbl)[])  [unwired: 7 in]
              n66 = call "add_waveforms.vi"("Error in (no error)"=w433, "Waveform array"=w430) -> ("Error out"=w428:errorcluster, "Summed waveform"=w431:waveform(dbl))  [unwired: 8 in]
              n67 = Array Size(array=w430) -> (size(s)=w429:i32)
              n68 = Divide(x=w431, y=w429) -> (x/y=→"Channel 1 RT avg":waveform(dbl))
            }
          }
          frame 1 {
            n69 = local read "Num Trace"() -> (w442:dbl)
            n70 = Get Queue Status(queue=w444, error in (no error)=w445) -> (queue out=w440:refnum<queue>, error out=w439:errorcluster, # elements in queue=w441:i32)  [unwired: 1 in, 5 out]
            n71 = Equal?(x=w441, y=w442) -> (x = y?=w443:bool)
            n72 = case shown="True" w443 {
              tunnel: w440 -> [w455 w476]
              tunnel: w439 -> [w454 w475]
              tunnel: [w446 w461] -> w438
              frame False {
                n73 = Get Queue Status(queue=w455, error in (no error)=w454) -> (error out=w448:errorcluster, elements=w449:waveform(dbl)[])  [unwired: 1 in, 6 out]
                n74 = call-poly <vilib>:"Align Waveform Timestamps.vi"("error in (no error)"=w448, "index"=0, "waveforms in"=w449) -> ("error out"=w453:errorcluster, "waveforms out"=w452:waveform(dbl)[])  [unwired: 7 in]
                n75 = call "add_waveforms.vi"("Error in (no error)"=w453, "Waveform array"=w452) -> ("Summed waveform"=w447:waveform(dbl))  [unwired: 8 in, 1 out]
                n76 = Array Size(array=w452) -> (size(s)=w450:i32)
                n77 = Divide(x=w447, y=w450) -> (x/y=w446:waveform(dbl))
              }
              frame True {
                n78 = Current VI's Path() -> (path=w467:path)
                n79 = Flush Queue(queue=w476, error in (no error)=w475) -> (remaining elements=w471:waveform(dbl)[], error out=w468:errorcluster)  [unwired: 1 out]
                n80 = Path To String(path=w467) -> (string=w458:string)
                n81 = xnode "Match Regular Expression"("input string"=w458, "regular expression"="scope_viewer") -> ("before match"=w456:string)  [unwired: 4 in, 4 out]
                n82 = call-poly <vilib>:"Align Waveform Timestamps.vi"("error in (no error)"=w468, "index"=0, "waveforms in"=w471) -> ("error out"=w474:errorcluster, "waveforms out"=w473:waveform(dbl)[])  [unwired: 7 in]
                n83 = call "add_waveforms.vi"("Error in (no error)"=w474, "Waveform array"=w473) -> ("Error out"=w463:errorcluster, "Summed waveform"=w470:waveform(dbl))  [unwired: 8 in]
                n84 = Array Size(array=w473) -> (size(s)=w469:i32)
                n85 = Concatenate Strings(w456, "\\summed_wfm_C1.csv" ("string")) -> (w466:string)
                n86 = String To Path(string=w466) -> (path=w459:path)
                n87 = Divide(x=w470, y=w469) -> (x/y=w461:waveform(dbl))
                n88 = call-poly <vilib>:"Export Waveforms to Spreadsheet File.vi"("header? (write header:T)"=TRUE, "delimiter (Tab)"=",", "append to file? (new file:F)"=FALSE, "error in (no error)"=w463, "waveform"=w461, "file path (dialog if empty)"=w459) -> ()  [unwired: 4 in, 2 out]
              }
            }
            "Channel 1 summed" <- w438
          }
        }
      }
    }
    n89 = case shown="True" w242 {
      tunnel: w244 -> [w248 w250]
      tunnel: w240 -> [w247 w249]
      tunnel: "Summed/Average" -> [_ w251]
      frame False {
        n90 = Flush Queue(queue=w248, error in (no error)=w247) -> ()  [unwired: 3 out]
      }
      frame True {
        n91 = case shown="1" w251 {
          tunnel: w250 -> [w253 w272]
          tunnel: w249 -> [w252 w273]
          frame 0, Default {
            # "Average"
            n92 = while {
              tunnel: w253 -> [w265]
              tunnel: w252 -> [w264]
              stop <- w256 stop-if-true
              n93 = Get Queue Status(queue=w265, return elements? (F)=TRUE, error in (no error)=w264) -> (error out=w262:errorcluster, elements=w263:waveform(dbl)[])  [unwired: 6 out]
              n94 = call-poly <vilib>:"Align Waveform Timestamps.vi"("error in (no error)"=w262, "index"=0, "waveforms in"=w263) -> ("error out"=w261:errorcluster, "waveforms out"=w258:waveform(dbl)[])  [unwired: 7 in]
              n95 = call "add_waveforms.vi"("Error in (no error)"=w261, "Waveform array"=w258) -> ("Error out"=w256:errorcluster, "Summed waveform"=w259:waveform(dbl))  [unwired: 8 in]
              n96 = Array Size(array=w258) -> (size(s)=w257:i32)
              n97 = Divide(x=w259, y=w257) -> (x/y=→"Channel 2 RT avg":waveform(dbl))
            }
          }
          frame 1 {
            n98 = local read "Num Trace"() -> (w267:dbl)
            n99 = Get Queue Status(queue=w272, error in (no error)=w273) -> (queue out=w269:refnum<queue>, error out=w268:errorcluster, # elements in queue=w270:i32)  [unwired: 1 in, 5 out]
            n100 = Equal?(x=w270, y=w267) -> (x = y?=w271:bool)
            n101 = case shown="True" w271 {
              tunnel: w269 -> [w283 w304]
              tunnel: w268 -> [w282 w303]
              tunnel: [w274 w289] -> w266
              frame False {
                n102 = Get Queue Status(queue=w283, error in (no error)=w282) -> (error out=w276:errorcluster, elements=w277:waveform(dbl)[])  [unwired: 1 in, 6 out]
                n103 = call-poly <vilib>:"Align Waveform Timestamps.vi"("error in (no error)"=w276, "index"=0, "waveforms in"=w277) -> ("error out"=w281:errorcluster, "waveforms out"=w280:waveform(dbl)[])  [unwired: 7 in]
                n104 = call "add_waveforms.vi"("Error in (no error)"=w281, "Waveform array"=w280) -> ("Summed waveform"=w275:waveform(dbl))  [unwired: 8 in, 1 out]
                n105 = Array Size(array=w280) -> (size(s)=w278:i32)
                n106 = Divide(x=w275, y=w278) -> (x/y=w274:waveform(dbl))
              }
              frame True {
                n107 = Current VI's Path() -> (path=w288:path)
                n108 = Flush Queue(queue=w304, error in (no error)=w303) -> (remaining elements=w299:waveform(dbl)[], error out=w296:errorcluster)  [unwired: 1 out]
                n109 = Path To String(path=w288) -> (string=w287:string)
                n110 = xnode "Match Regular Expression"("input string"=w287, "regular expression"="scope_viewer") -> ("before match"=w285:string)  [unwired: 4 in, 4 out]
                n111 = call-poly <vilib>:"Align Waveform Timestamps.vi"("error in (no error)"=w296, "index"=0, "waveforms in"=w299) -> ("error out"=w302:errorcluster, "waveforms out"=w301:waveform(dbl)[])  [unwired: 7 in]
                n112 = Concatenate Strings(w285, "\\summed_wfm_C2.csv" ("string")) -> (w295:string)
                n113 = String To Path(string=w295) -> (path=w293:path)
                n114 = call "add_waveforms.vi"("Error in (no error)"=w302, "Waveform array"=w301) -> ("Error out"=w291:errorcluster, "Summed waveform"=w298:waveform(dbl))  [unwired: 8 in]
                n115 = Array Size(array=w301) -> (size(s)=w297:i32)
                n116 = Divide(x=w298, y=w297) -> (x/y=w289:waveform(dbl))
                n117 = call-poly <vilib>:"Export Waveforms to Spreadsheet File.vi"("header? (write header:T)"=TRUE, "delimiter (Tab)"=",", "append to file? (new file:F)"=FALSE, "error in (no error)"=w291, "waveform"=w289, "file path (dialog if empty)"=w293) -> ()  [unwired: 4 in, 2 out]
              }
            }
            "Channel 2 summed" <- w266
          }
        }
      }
    }
    n118 = Or(x=w240, y=w239) -> (x .or. y?=w241:bool)
  }
  n119 = Current VI's Path() -> (path=w23:path)
  n120 = while {
    shift-right: [w596] -> _
    shift-left: w20 -> [w597]
    shift-right: [w593] -> _
    shift-left: w23 -> [w594]
    tunnel: w19 -> [w592]
    tunnel: w18 -> [w591]
    stop <- w595 stop-if-true
    n121 = event shown="[17] \"tmax (\\mu s)\": Value Change" {
      selector: _ -> [_ _ _ _ _ _ _ _ _ _ _ _ _ _ _ _ _ _ _ _ _ _ _ _ _]
      dyn-events: _ -> [_ _ _ _ _ _ _ _ _ _ _ _ _ _ _ _ _ _ _ _ _ _ _ _ _]
      timeout: _ -> [_ _ _ _ _ _ _ _ _ _ _ _ _ _ _ _ _ _ _ _ _ _ _ _ _]
      tunnel: w597 -> [w603 w610 w617 w631 w642 w653 w664 w675 w686 w698 w709 w718 w726 w734 w742 w744 w755 w766 w777 w787 w797 w807 w817 w826 w862]
      tunnel: [w601 w610 w615 w630 w641 w652 w663 w674 w685 w697 w708 w717 w725 w733 w741 w744 w755 w766 w777 w787 w797 w807 w817 w826 w859] -> w596
      tunnel: [_ w611 _ _ _ _ _ _ _ _ _ _ _ _ _ _ _ _ _ _ _ _ _ _ _] -> w595
      tunnel: w594 -> [w598 w609 w612 w623 w634 w645 w656 w667 w678 w689 w700 w711 w719 w727 w735 w743 w754 w765 w776 w786 w796 w806 w816 w827 w863]
      tunnel: [w598 w609 w612 w623 w634 w645 w656 w667 w678 w689 w700 w711 w719 w727 w735 w743 w754 w765 w776 w786 w796 w806 w816 w828 w836] -> w593
      tunnel: w592 -> [w600 _ w614 w625 w636 w647 w658 w669 w680 w693 w704 w713 w721 w729 w737 w746 w757 w768 w779 w789 w799 w809 w819 _ w861]
      tunnel: w591 -> [w599 _ w613 w624 w635 w646 w657 w668 w679 w692 w703 w712 w720 w728 w736 w745 w756 w767 w778 w788 w798 w808 w818 _ w860]
      event "C1 vertical offset": Value Change {
        n122 = event-data() -> ("NewVal"=w602:dbl)  [unwired: 1 in, 5 out]
        n123 = Unbundle By Name(w603) -> ("C1 vertical range"=w607:dbl, "C1 probe attenuation"=w605:dbl, "C1 vertical coupling"=w608:T2, "C1 enabled"=w606:bool)
        n124 = call <instrlib>:"niScope Configure Vertical.vi"("instrument handle"=w600, "probe attenuation"=w605, "vertical coupling"=w608, "channels"="0", "vertical range"=w607, "vertical offset"=w602, "error in"=w599, "channel enabled"=w606) -> ()  [unwired: 6 in, 2 out]
        n125 = Bundle By Name(cluster=w603, "C1 vertical offset"=w602) -> (w601:T7)
      }
      event "stop": Value Change {
        n126 = event-data() -> ("NewVal"=w611:bool)  [unwired: 1 in, 5 out]
      }
      event "C2 vertical offset": Value Change {
        n127 = event-data() -> ("NewVal"=w616:dbl)  [unwired: 1 in, 5 out]
        n128 = Unbundle By Name(w617) -> ("C2 vertical range"=w621:dbl, "C2 probe attenuation"=w619:dbl, "C2 probe attenuation"=w622:dbl, "C2 enabled"=w620:bool)
        n129 = call <instrlib>:"niScope Configure Vertical.vi"("instrument handle"=w614, "probe attenuation"=w619, "vertical coupling"=w622, "channels"="1", "vertical range"=w621, "vertical offset"=w616, "error in"=w613, "channel enabled"=w620) -> ()  [unwired: 6 in, 2 out]
        n130 = Bundle By Name(cluster=w617, "C2 vertical offset"=w616) -> (w615:T7)
      }
      event "C1 vertical range": Value Change {
        n131 = event-data() -> ("NewVal"=w626:dbl)  [unwired: 1 in, 5 out]
        n132 = Unbundle By Name(w631) -> ("C1 vertical offset"=w629:dbl, "C1 probe attenuation"=w628:dbl, "C1 vertical coupling"=w627:T2, "C1 enabled"=w633:bool)
        n133 = call <instrlib>:"niScope Configure Vertical.vi"("instrument handle"=w625, "probe attenuation"=w628, "vertical coupling"=w627, "channels"="0", "vertical range"=w626, "vertical offset"=w629, "error in"=w624, "channel enabled"=w633) -> ()  [unwired: 6 in, 2 out]
        n134 = Bundle By Name(cluster=w631, "C1 vertical range"=w626) -> (w630:T7)
      }
      event "C2 vertical range": Value Change {
        n135 = event-data() -> ("NewVal"=w637:dbl)  [unwired: 1 in, 5 out]
        n136 = Unbundle By Name(w642) -> ("C2 vertical offset"=w640:dbl, "C2 probe attenuation"=w639:dbl, "C2 vertical coupling"=w638:T2, "C2 enabled"=w644:bool)
        n137 = call <instrlib>:"niScope Configure Vertical.vi"("instrument handle"=w636, "probe attenuation"=w639, "vertical coupling"=w638, "channels"="1", "vertical range"=w637, "vertical offset"=w640, "error in"=w635, "channel enabled"=w644) -> ()  [unwired: 6 in, 2 out]
        n138 = Bundle By Name(cluster=w642, "C2 vertical range"=w637) -> (w641:T7)
      }
      event "C1 probe attenuation": Value Change {
        n139 = event-data() -> ("NewVal"=w648:dbl)  [unwired: 1 in, 5 out]
        n140 = Unbundle By Name(w653) -> ("C1 vertical offset"=w651:dbl, "C1 vertical range"=w650:dbl, "C1 vertical coupling"=w649:T2, "C1 enabled"=w655:bool)
        n141 = call <instrlib>:"niScope Configure Vertical.vi"("instrument handle"=w647, "probe attenuation"=w648, "vertical coupling"=w649, "channels"="0", "vertical range"=w650, "vertical offset"=w651, "error in"=w646, "channel enabled"=w655) -> ()  [unwired: 6 in, 2 out]
        n142 = Bundle By Name(cluster=w653, "C1 probe attenuation"=w648) -> (w652:T7)
      }
      event "C2 probe attenuation": Value Change {
        n143 = event-data() -> ("NewVal"=w659:dbl)  [unwired: 1 in, 5 out]
        n144 = Unbundle By Name(w664) -> ("C2 vertical offset"=w662:dbl, "C2 vertical range"=w661:dbl, "C2 vertical coupling"=w660:T2, "C2 enabled"=w666:bool)
        n145 = call <instrlib>:"niScope Configure Vertical.vi"("instrument handle"=w658, "probe attenuation"=w659, "vertical coupling"=w660, "channels"="1", "vertical range"=w661, "vertical offset"=w662, "error in"=w657, "channel enabled"=w666) -> ()  [unwired: 6 in, 2 out]
        n146 = Bundle By Name(cluster=w664, "C2 probe attenuation"=w659) -> (w663:T7)
      }
      event Value Change {
        n147 = event-data() -> ("NewVal"=w671:T2)  [unwired: 1 in, 5 out]
        n148 = Unbundle By Name(w675) -> ("C1 vertical offset"=w673:dbl, "C1 vertical range"=w672:dbl, "C1 probe attenuation"=w670:dbl, "C1 enabled"=w677:bool)
        n149 = call <instrlib>:"niScope Configure Vertical.vi"("instrument handle"=w669, "probe attenuation"=w670, "vertical coupling"=w671, "channels"="0", "vertical range"=w672, "vertical offset"=w673, "error in"=w668, "channel enabled"=w677) -> ()  [unwired: 6 in, 2 out]
        n150 = Bundle By Name(cluster=w675, "C1 vertical coupling"=w671) -> (w674:T7)
      }
      event Value Change {
        n151 = event-data() -> ("NewVal"=w682:T2)  [unwired: 1 in, 5 out]
        n152 = Unbundle By Name(w686) -> ("C2 vertical offset"=w684:dbl, "C2 vertical range"=w683:dbl, "C2 probe attenuation"=w681:dbl, "C2 enabled"=w688:bool)
        n153 = call <instrlib>:"niScope Configure Vertical.vi"("instrument handle"=w680, "probe attenuation"=w681, "vertical coupling"=w682, "channels"="1", "vertical range"=w683, "vertical offset"=w684, "error in"=w679, "channel enabled"=w688) -> ()  [unwired: 6 in, 2 out]
        n154 = Bundle By Name(cluster=w686, "C2 vertical coupling"=w682) -> (w685:T7)
      }
      event "C1 enabled": Value Change {
        n155 = event-data() -> ("NewVal"=w695:bool)  [unwired: 1 in, 5 out]
        n156 = Unbundle By Name(w698) -> ("C1 vertical offset"=w690:dbl, "C1 vertical range"=w691:dbl, "C1 probe attenuation"=w696:dbl, "C1 vertical coupling"=w694:T2)
        n157 = call <instrlib>:"niScope Configure Vertical.vi"("instrument handle"=w693, "probe attenuation"=w696, "vertical coupling"=w694, "channels"="0", "vertical range"=w691, "vertical offset"=w690, "error in"=w692, "channel enabled"=w695) -> ()  [unwired: 6 in, 2 out]
        n158 = Bundle By Name(cluster=w698, "C1 enabled"=w695) -> (w697:T7)
      }
      event "C2 enabled": Value Change {
        n159 = event-data() -> ("NewVal"=w706:bool)  [unwired: 1 in, 5 out]
        n160 = Unbundle By Name(w709) -> ("C2 vertical offset"=w701:dbl, "C2 vertical range"=w702:dbl, "C2 probe attenuation"=w707:dbl, "C2 vertical coupling"=w705:T2)
        n161 = call <instrlib>:"niScope Configure Vertical.vi"("instrument handle"=w704, "probe attenuation"=w707, "vertical coupling"=w705, "channels"="1", "vertical range"=w702, "vertical offset"=w701, "error in"=w703, "channel enabled"=w706) -> ()  [unwired: 6 in, 2 out]
        n162 = Bundle By Name(cluster=w709, "C2 enabled"=w706) -> (w708:T7)
      }
      event "C1 maximum input frequency": Value Change {
        n163 = event-data() -> ("NewVal"=w714:dbl)  [unwired: 1 in, 5 out]
        n164 = Unbundle By Name(w718) -> ("C1 input impedance"=w715:u32)
        n165 = Bundle By Name(cluster=w718, "C1 maximum input frequency"=w714) -> (w717:T7)
        n166 = call <instrlib>:"niScope Configure Chan Characteristics.vi"("instrument handle"=w713, "channels"="0", "input impedance"=w715, "maximum input frequency"=w714, "error in"=w712) -> ()  [unwired: 9 in, 2 out]
      }
      event "C2 maximum input frequency": Value Change {
        n167 = event-data() -> ("NewVal"=w722:dbl)  [unwired: 1 in, 5 out]
        n168 = Unbundle By Name(w726) -> ("C2 input impedance"=w723:u32)
        n169 = Bundle By Name(cluster=w726, "C2 maximum input frequency"=w722) -> (w725:T7)
        n170 = call <instrlib>:"niScope Configure Chan Characteristics.vi"("instrument handle"=w721, "channels"="1", "input impedance"=w723, "maximum input frequency"=w722, "error in"=w720) -> ()  [unwired: 9 in, 2 out]
      }
      event "C1 input impedance": Value Change {
        n171 = event-data() -> ("NewVal"=w731:u32)  [unwired: 1 in, 5 out]
        n172 = Unbundle By Name(w734) -> ("C1 maximum input frequency"=w730:dbl)
        n173 = Bundle By Name(cluster=w734, "C1 input impedance"=w731) -> (w733:T7)
        n174 = call <instrlib>:"niScope Configure Chan Characteristics.vi"("instrument handle"=w729, "channels"="0", "input impedance"=w731, "maximum input frequency"=w730, "error in"=w728) -> ()  [unwired: 9 in, 2 out]
      }
      event "C2 input impedance": Value Change {
        n175 = event-data() -> ("NewVal"=w739:u32)  [unwired: 1 in, 5 out]
        n176 = Unbundle By Name(w742) -> ("C2 maximum input frequency"=w738:dbl)
        n177 = Bundle By Name(cluster=w742, "C2 input impedance"=w739) -> (w741:T7)
        n178 = call <instrlib>:"niScope Configure Chan Characteristics.vi"("instrument handle"=w737, "channels"="1", "input impedance"=w739, "maximum input frequency"=w738, "error in"=w736) -> ()  [unwired: 9 in, 2 out]
      }
      event "Enforce realtime": Value Change {
        n179 = event-data() -> ("NewVal"=w753:bool)  [unwired: 1 in, 5 out]
        n180 = Unbundle By Name(w744) -> ("Samples"=w751:i64, "tmax (\\mu s)"=w749:dbl)
        n181 = call "set_sample_rate.vi"("t max / us"=w749, "Samples"=w751) -> ("Min sample rate"=w747:dbl, "Min record length"=w750:dbl)  [unwired: 8 in]
        n182 = Bundle By Name(cluster=w744, "Enforce realtime"=w753) -> ()  [unwired: 1 out]
        n183 = call <instrlib>:"niScope Configure Horizontal Timing.vi"("instrument handle"=w746, "number of records"=1, "enforce realtime"=w753, "min sample rate"=w747, "reference position"=0.0, "error in"=w745, "min record length"=w750) -> ()  [unwired: 7 in, 2 out]
      }
      event "Samples": Value Change {
        n184 = event-data() -> ("NewVal"=w759:i64)  [unwired: 1 in, 5 out]
        n185 = Unbundle By Name(w755) -> ("Enforce realtime"=w758:bool, "tmax (\\mu s)"=w762:dbl)
        n186 = call "set_sample_rate.vi"("t max / us"=w762, "Samples"=w759) -> ("Min sample rate"=w760:dbl, "Min record length"=w763:dbl)  [unwired: 8 in]
        n187 = Bundle By Name(cluster=w755, "Samples"=w759) -> ()  [unwired: 1 out]
        n188 = call <instrlib>:"niScope Configure Horizontal Timing.vi"("instrument handle"=w757, "number of records"=1, "enforce realtime"=w758, "min sample rate"=w760, "reference position"=0.0, "error in"=w756, "min record length"=w763) -> ()  [unwired: 7 in, 2 out]
      }
      event "tmax (\\mu s)": Value Change {
        n189 = event-data() -> ("NewVal"=w769:dbl)  [unwired: 1 in, 5 out]
        n190 = Unbundle By Name(w766) -> ("Enforce realtime"=w771:bool, "Samples"=w770:i64)
        n191 = call "set_sample_rate.vi"("t max / us"=w769, "Samples"=w770) -> ("Min sample rate"=w772:dbl, "Min record length"=w774:dbl)  [unwired: 8 in]
        n192 = Bundle By Name(cluster=w766, "tmax (\\mu s)"=w769) -> ()  [unwired: 1 out]
        n193 = call <instrlib>:"niScope Configure Horizontal Timing.vi"("instrument handle"=w768, "number of records"=1, "enforce realtime"=w771, "min sample rate"=w772, "reference position"=0.0, "error in"=w767, "min record length"=w774) -> ()  [unwired: 7 in, 2 out]
      }
      event Value Change {
        n194 = event-data() -> ("NewVal"=w780:T5)  [unwired: 1 in, 5 out]
        n195 = Unbundle By Name(w777) -> ("Trigger coupling"=w785:T4, "Trigger level"=w783:dbl, "Trigger slope"=w784:T3, "Trigger delay"=w781:dbl)
        n196 = call-poly <instrlib>:"niScope Configure Trigger (poly).vi"("instrument handle"=w779, "trigger slope"=w784, "trigger coupling"=w785, "trigger source"=w780, "trigger level"=w783, "error in"=w778, "trigger holdoff"=0.0, "trigger delay"=w781) -> ()  [unwired: 6 in, 2 out]
        n197 = Bundle By Name(cluster=w777, "Trigger source"=w780) -> ()  [unwired: 1 out]
      }
      event Value Change {
        n198 = event-data() -> ("NewVal"=w790:T4)  [unwired: 1 in, 5 out]
        n199 = Unbundle By Name(w787) -> ("Trigger source"=w791:T5, "Trigger level"=w794:dbl, "Trigger slope"=w795:T3, "Trigger delay"=w792:dbl)
        n200 = call-poly <instrlib>:"niScope Configure Trigger (poly).vi"("instrument handle"=w789, "trigger slope"=w795, "trigger coupling"=w790, "trigger source"=w791, "trigger level"=w794, "error in"=w788, "trigger holdoff"=0.0, "trigger delay"=w792) -> ()  [unwired: 6 in, 2 out]
        n201 = Bundle By Name(cluster=w787, "Trigger coupling"=w790) -> ()  [unwired: 1 out]
      }
      event "Trigger level": Value Change {
        n202 = event-data() -> ("NewVal"=w800:dbl)  [unwired: 1 in, 5 out]
        n203 = Unbundle By Name(w797) -> ("Trigger source"=w802:T5, "Trigger coupling"=w801:T4, "Trigger slope"=w805:T3, "Trigger delay"=w803:dbl)
        n204 = call-poly <instrlib>:"niScope Configure Trigger (poly).vi"("instrument handle"=w799, "trigger slope"=w805, "trigger coupling"=w801, "trigger source"=w802, "trigger level"=w800, "error in"=w798, "trigger holdoff"=0.0, "trigger delay"=w803) -> ()  [unwired: 6 in, 2 out]
        n205 = Bundle By Name(cluster=w797, "Trigger level"=w800) -> ()  [unwired: 1 out]
      }
      event Value Change {
        n206 = event-data() -> ("NewVal"=w811:T3)  [unwired: 1 in, 5 out]
        n207 = Unbundle By Name(w807) -> ("Trigger source"=w813:T5, "Trigger coupling"=w812:T4, "Trigger level"=w810:dbl, "Trigger delay"=w814:dbl)
        n208 = call-poly <instrlib>:"niScope Configure Trigger (poly).vi"("instrument handle"=w809, "trigger slope"=w811, "trigger coupling"=w812, "trigger source"=w813, "trigger level"=w810, "error in"=w808, "trigger holdoff"=0.0, "trigger delay"=w814) -> ()  [unwired: 6 in, 2 out]
        n209 = Bundle By Name(cluster=w807, "Trigger slope"=w811) -> ()  [unwired: 1 out]
      }
      event "Trigger delay": Value Change {
        n210 = event-data() -> ("NewVal"=w821:dbl)  [unwired: 1 in, 5 out]
        n211 = Unbundle By Name(w817) -> ("Trigger source"=w824:T5, "Trigger coupling"=w823:T4, "Trigger level"=w822:dbl, "Trigger slope"=w820:T3)
        n212 = call-poly <instrlib>:"niScope Configure Trigger (poly).vi"("instrument handle"=w819, "trigger slope"=w820, "trigger coupling"=w823, "trigger source"=w824, "trigger level"=w822, "error in"=w818, "trigger holdoff"=0.0, "trigger delay"=w821) -> ()  [unwired: 6 in, 2 out]
        n213 = Bundle By Name(cluster=w817, "Trigger delay"=w821) -> ()  [unwired: 1 out]
      }
      event "Save Scope Conditions": Value Change {
        n214 = event-data() -> ()  [unwired: 1 in, 6 out]
        n215 = call "File Dialog"("start path"=w827) -> ("selected path"=w829:path, "error out"=w830:errorcluster)  [unwired: 11 in, 2 out]
        n216 = case shown="No Error" w830 {
          selector: w830 -> [w832 w835]
          tunnel: w829 -> [w831 _]
          tunnel: w826 -> [w833 _]
          tunnel: [w831 w834] -> w828
          tunnel: w827 -> [_ w834]
          frame No Error {
            n217 = Write to Binary File(file (use dialog)=w831, data=w833, error in=w832) -> ()  [unwired: 3 in, 3 out]
          }
          frame Error {
            n218 = call "Display Message to User"("error in (no error)"=w835) -> ()  [unwired: 9 in, 2 out]
          }
        }
      }
      event "Load Scope Conditions": Value Change {
        n219 = event-data() -> ()  [unwired: 1 in, 6 out]
        n220 = call "Load File Dialogue"("start path"=w863) -> ("selected path"=w836:path)  [unwired: 11 in, 3 out]
        n221 = Read from Binary File(5:w862, 11:w836) -> (2:w859:T7)  [unwired: 4 in, 3 out]
        n222 = Unbundle By Name(w859) -> ("C2 vertical offset"=w858:dbl, "C2 vertical range"=w857:dbl, "C2 probe attenuation"=w856:dbl, "C2 vertical coupling"=w855:T2, "C2 maximum input frequency"=w854:dbl, "C2 input impedance"=w853:u32, "C2 enabled"=w852:bool, "C1 input impedance"=w851:u32, "C1 maximum input frequency"=w850:dbl, "C1 enabled"=w849:bool, "C1 vertical offset"=w848:dbl, "C1 vertical range"=w847:dbl, "C1 probe attenuation"=w846:dbl, "C1 vertical coupling"=w845:T2, "Samples"=w844:i64, "tmax (\\mu s)"=w843:dbl, "Trigger source"=w842:T5, "Trigger coupling"=w841:T4, "Trigger level"=w840:dbl, "Trigger slope"=w839:T3, "Trigger delay"=w838:dbl, "Enforce realtime"=w837:bool)
        n223 = call "config_scope.vi"("instrument handle"=w861, "Scope Config Data"=w859, "error in"=w860) -> ()  [unwired: 11 in, 2 out]
        n224 = local write "C2 vertical offset"(w858) -> ()
        n225 = local write "C2 vertical range"(w857) -> ()
        n226 = local write "C2 probe attenuation"(w856) -> ()
        n227 = local write "C2 vertical coupling"(w855) -> ()
        n228 = local write "C2 maximum input frequency"(w854) -> ()
        n229 = local write "C2 input impedance"(w853) -> ()
        n230 = local write "C2 enabled"(w852) -> ()
        n231 = local write "C1 input impedance"(w851) -> ()
        n232 = local write "C1 maximum input frequency"(w850) -> ()
        n233 = local write "C1 enabled"(w849) -> ()
        n234 = local write "C1 vertical range"(w847) -> ()
        n235 = local write "C1 probe attenuation"(w846) -> ()
        n236 = local write "C1 vertical coupling"(w845) -> ()
        n237 = local write "tmax (\\mu s)"(w843) -> ()
        n238 = local write "C1 vertical offset"(w848) -> ()
        n239 = local write "Samples"(w844) -> ()
        n240 = local write "Trigger source"(w842) -> ()
        n241 = local write "Trigger coupling"(w841) -> ()
        n242 = local write "Trigger level"(w840) -> ()
        n243 = local write "Trigger slope"(w839) -> ()
        n244 = local write "Trigger delay"(w838) -> ()
        n245 = local write "Enforce realtime"(w837) -> ()
      }
    }
  }
  n246 = call <instrlib>:"niScope Close.vi"("instrument handle"=w64, "error in"=w63) -> ()  [unwired: 13 in, 1 out]
